vi "new.vi"(8 "error in (no error)":errorcluster, 11 "data":dbl) -> (0 "error out":errorcluster, 3 "DoublyNodeRef out":refnum<class "DoublyNodeRef.lvclass">)   [LabVIEW 2021, in "DoublyNodeRef.lvclass"]
uses:
  DoublyNodeRef.lvclass
  DoublyNodeRef.lvclass/DoublyNodeRef.ctl
  IDoublyNode/IDoublyNode.lvclass
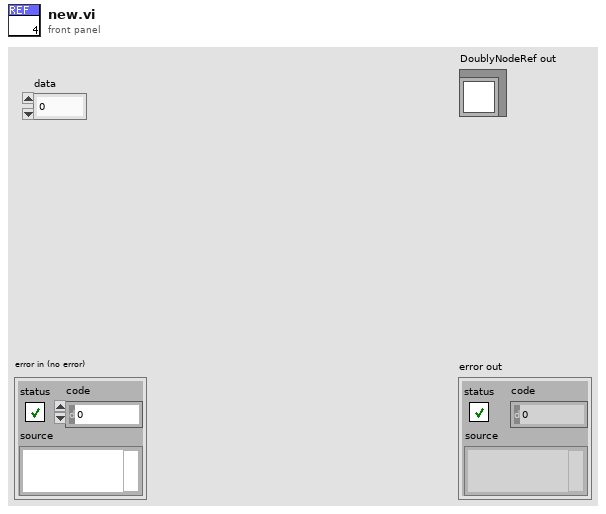
[diagram p1: front panel]
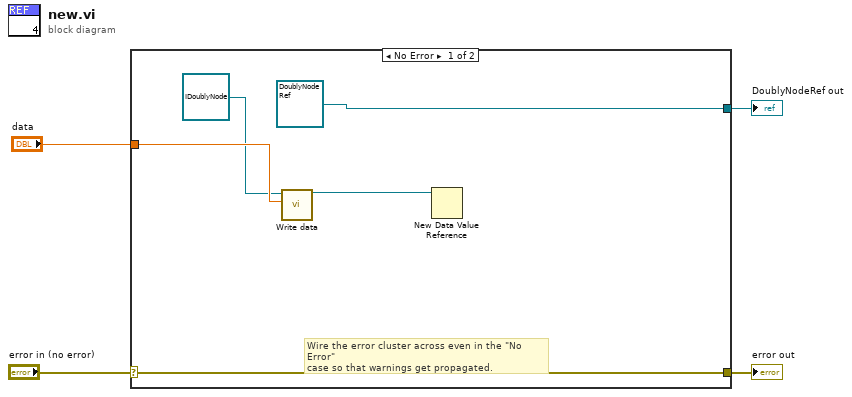
[diagram p0: block diagram]
diagram:
  n1 = case shown="No Error" "error in (no error)" {
    selector: "error in (no error)" -> [w9 w10]
    tunnel: [w9 w10] -> w3
    tunnel: [refnum<class "DoublyNodeRef.lvclass"> refnum ("DoublyNodeRef out") _] -> w2
    tunnel: "data" -> [w7 _]
    frame No Error {
      # "Wire the error cluster across even in the \"No Error\"\ncase so that warnings get propagated."
      n2 = call-dynamic "Write data.vi"("data"=w7, "IDoublyNode in"=refnum<class "IDoublyNode.lvclass"> refnum) -> ("IDoublyNode out"=w5:refnum<class "IDoublyNode.lvclass">)  [unwired: 8 in, 1 out]
      n3 = New Data Value Reference(data value=w5) -> ()  [unwired: 1 in, 2 out]
    }
    frame Error {
    }
  }
  "error out" <- w3
  "DoublyNodeRef out" <- w2
